vi "My First VI.vi"() -> ()   [LabVIEW 2020]
panel:
  out "Area of a triangle":dbl
  in  "Height":dbl
  in  "Base":dbl
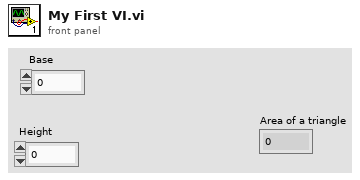
[diagram p1: front panel]
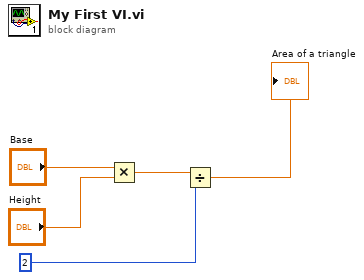
[diagram p0: block diagram]
diagram:
  n1 = Multiply(x="Base", y="Height") -> (x*y=w3:dbl)
  n2 = Divide(x=w3, y=2) -> (x/y=→"Area of a triangle":dbl)
